vi "Device.OnInitialized.vi"(8 "error in (no error)":errorcluster, 10 "Result":T1, 11 "Device in":refnum<class "Device.lvclass">) -> (0 "error out":errorcluster, 3 "Device out":refnum<class "Device.lvclass">)   [LabVIEW 2017, in "Device.lvclass"]
uses:
  Device.lvclass
  Typedefs/PublicEvents--Device.Initialized.ctl
  Device.lvclass/Device.ctl
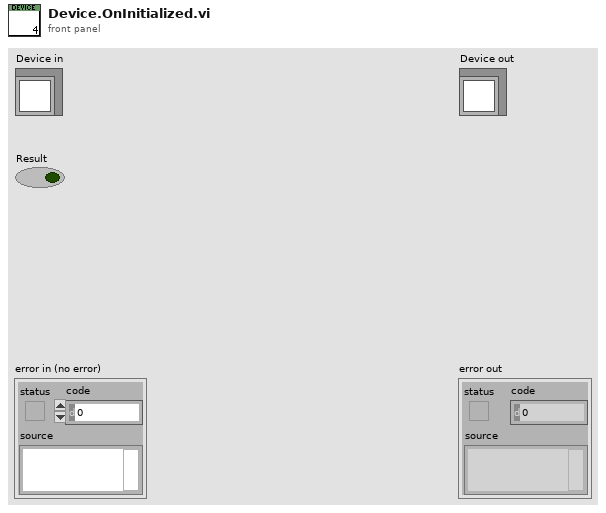
[diagram p1: front panel]
types:
  T1 = typedef "Device.lvclass/PublicEvents--Device.Initialized.ctl" = bool
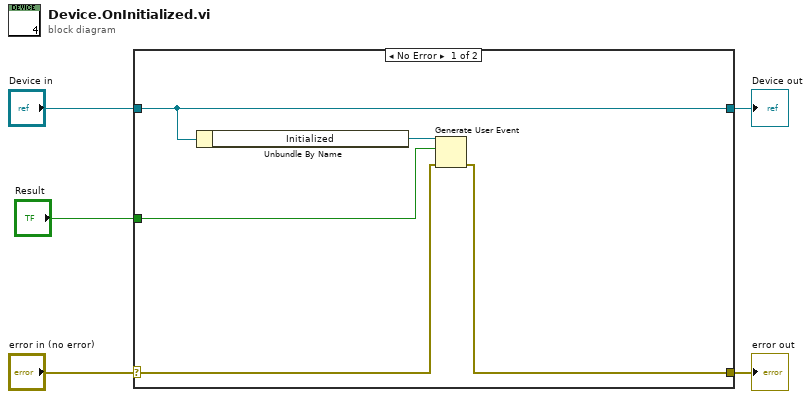
[diagram p0: block diagram]
diagram:
  n1 = case shown="No Error" "error in (no error)" {
    selector: "error in (no error)" -> [w7 w12]
    tunnel: [w6 w12] -> w4
    tunnel: [w10 w11] -> w2
    tunnel: "Device in" -> [w10 w11]
    tunnel: "Result" -> [w8 _]
    frame No Error {
      n2 = Unbundle By Name(w10) -> ("Initialized"=w9:refnum<user-event>)
      n3 = Generate User Event(user event=w9, event data cluster=w8, error in=w7) -> (error out=w6:errorcluster)  [unwired: 1 in, 1 out]
    }
    frame Error {
    }
  }
  "error out" <- w4
  "Device out" <- w2
